vi "Close My Data CSV.vi"(8 "error in":errorcluster, 11 "file refnum":refnum<file>) -> (0 "error out":errorcluster)   [LabVIEW 2014]
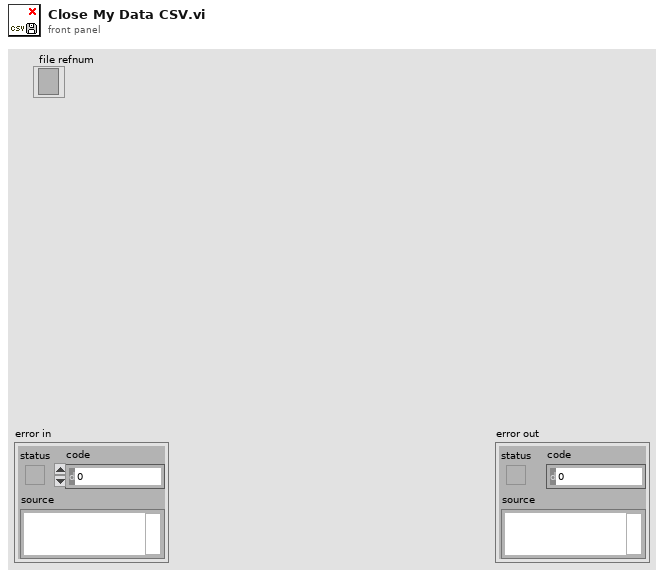
[diagram p1: front panel]
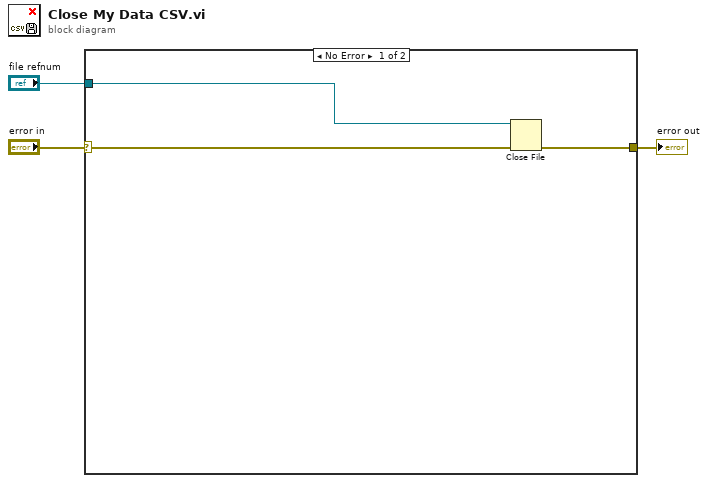
[diagram p0: block diagram]
diagram:
  n1 = case shown="No Error" "error in" {
    selector: "error in" -> [w5 w7]
    tunnel: [w6 w7] -> w3
    tunnel: "file refnum" -> [w4 _]
    frame No Error {
      n2 = Close File(refnum=w4, error in=w5) -> (error out=w6:errorcluster)  [unwired: 1 out]
    }
    frame Error {
      # "Wire previous error through"
    }
  }
  "error out" <- w3
